vi "harmony_final.vi"() -> ()   [LabVIEW 2017]
uses:
  <vilib>/measure/maspectr.llb/FFT Spectrum (Mag-Phase) for 1 Chan.vi
  <vilib>/Instr/_visa.llb/VISA Configure Serial Port (Instr).vi
  <vilib>/measure/NI_MAPro.lvlib
panel:
  out "Si":bool
  out "Lá":bool
  out "Sol":bool
  out "Fá":bool
  out "Mi":bool
  out "Ré":bool
  out "Dó":bool
  out "Frequências":cluster{"f0":dbl, "df":dbl, "magnitude":dbl[]}(graph)
  out "Frequência":i32
  out "Waveform Chart":waveform(dbl)(graph)
  in  "Reset":bool
  in  "Porta Serial":refnum<visa-resource-name>
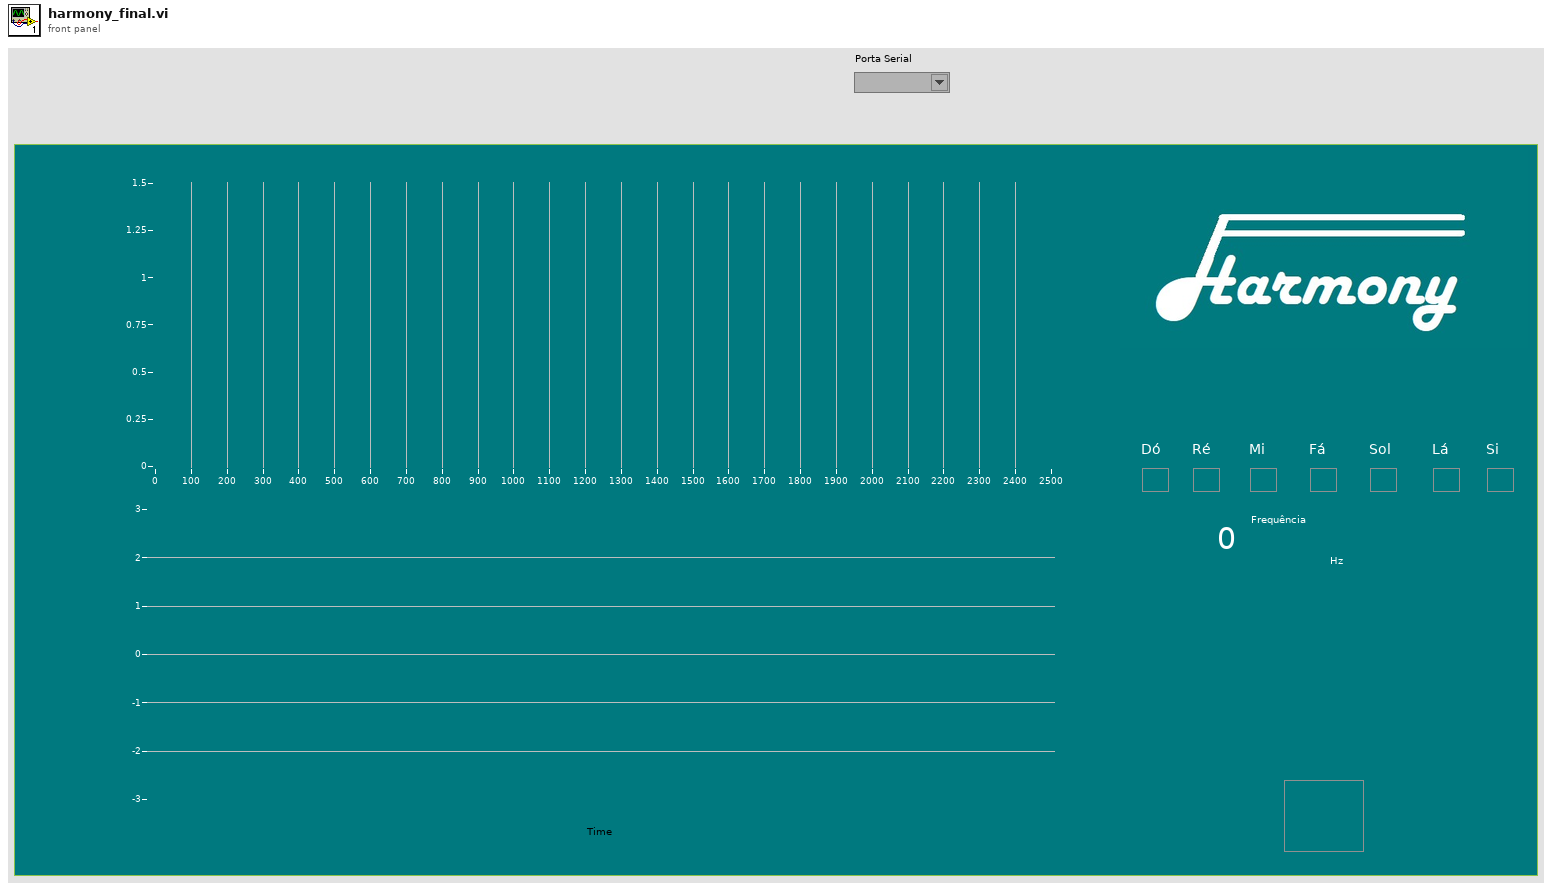
[diagram p1: front panel]
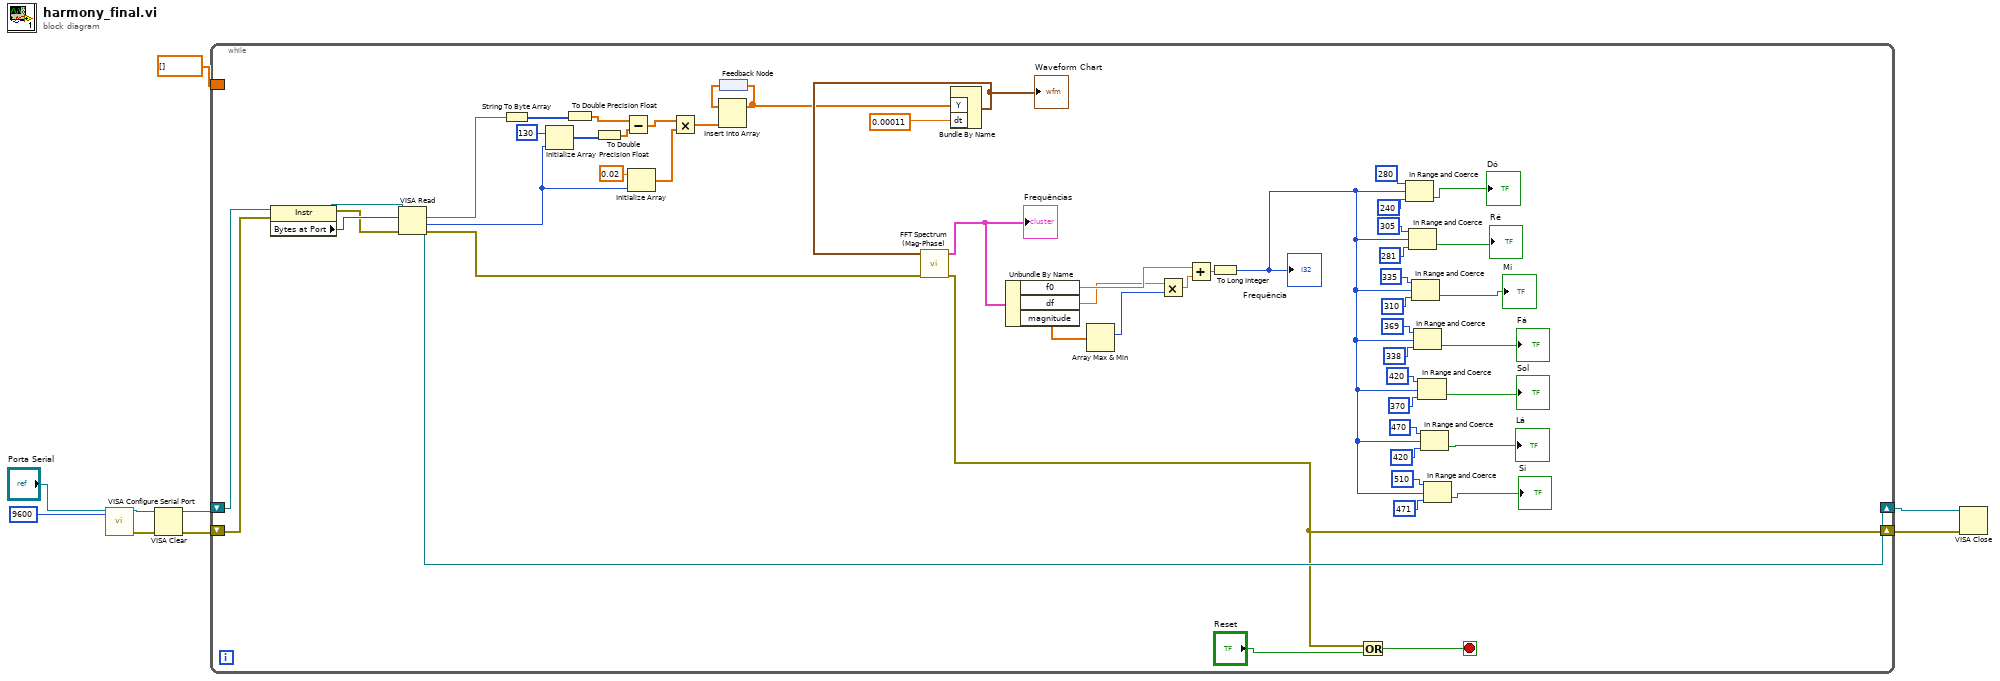
[diagram p0: block diagram]
diagram:
  n1 = call-poly "VISA Configure Serial Port"("VISA resource name"="Porta Serial", "baud rate (9600)"=u32 9600) -> ("VISA resource name out"=w7:refnum<visa-resource-name>, "error out"=w6:errorcluster)  [unwired: 12 in]
  n2 = VISA Clear(VISA resource name=w7, error in (no error)=w6) -> (VISA resource name out=w5:refnum<visa-resource-name>, error out=w4:errorcluster)
  n3 = while {
    shift-right: [w58] -> w3
    shift-left: w5 -> [w63]
    shift-right: [w34] -> w2
    shift-left: w4 -> [w62]
    border: dbl[] [] -> [_]
    stop <- w54 stop-if-true
    n4 = property class="Instr"(reference=w63, error in=w62) -> (reference out=w60:refnum<visa-resource-name>, error out=w59:errorcluster, "Bytes at Port"=w61:u32)
    n5 = VISA Read(VISA resource name=w60, byte count=w61, error in (no error)=w59) -> (VISA resource name out=w58:refnum<visa-resource-name>, read buffer=w56:string, return count=w44:u32, error out=w37:errorcluster)
    n6 = String To Byte Array(string=w56) -> (unsigned byte array=w51:u8[])
    n7 = Initialize Array(130, w44) -> (w46:i32[])
    n8 = To Double Precision Float(number=w51) -> (double precision float=w50:dbl[])
    n9 = To Double Precision Float(number=w46) -> (double precision float=w45:dbl[])
    n10 = Subtract(x=w50, y=w45) -> (x-y=w49:dbl[])
    n11 = Initialize Array(0.02, w44) -> (w42:dbl[])
    n12 = Multiply(x=w49, y=w42) -> (x*y=w48:dbl[])
    n13 = feedback #1() -> (w57:dbl[])
    n14 = Insert Into Array(array=w57, new element=w48) -> (w10:dbl[])  [unwired: 1 in]
    n15 = feedback-in #1(w10) -> ()
    n16 = Bundle By Name("Y"=w10, "dt"=0.00011) -> (w53:waveform(dbl))  [unwired: 1 in]
    "Waveform Chart" <- w53
    n17 = call-poly <vilib>:"FFT Spectrum (Mag-Phase).vi"("error in (no error)"=w37, "time signal"=w53) -> ("error out"=w34:errorcluster, "magnitude"=w52:cluster{"f0":dbl, "df":dbl, "magnitude":dbl[]})  [unwired: 5 in, 3 out]
    "Frequências" <- w52
    n18 = Unbundle By Name(w52) -> ("f0"=w39:dbl, "df"=w38:dbl, "magnitude"=w36:dbl[])
    n19 = Array Max & Min(array=w36) -> (max index (indices)=w35:i32)  [unwired: 3 out]
    n20 = Multiply(x=w38, y=w35) -> (x*y=w40:dbl)
    n21 = Add(x=w39, y=w40) -> (x+y=w41:dbl)
    n22 = To Long Integer(number=w41) -> (32bit integer=w18:i32)
    "Frequência" <- w18
    n23 = Or(x=w34, y="Reset") -> (x .or. y?=w54:bool)
    n24 = In Range and Coerce(upper limit=280, x=w18, lower limit=240) -> (In Range?=→"Dó":bool)  [unwired: 1 out]
    n25 = In Range and Coerce(upper limit=305, x=w18, lower limit=281) -> (In Range?=→"Ré":bool)  [unwired: 1 out]
    n26 = In Range and Coerce(upper limit=335, x=w18, lower limit=310) -> (In Range?=→"Mi":bool)  [unwired: 1 out]
    n27 = In Range and Coerce(upper limit=369, x=w18, lower limit=338) -> (In Range?=→"Fá":bool)  [unwired: 1 out]
    n28 = In Range and Coerce(upper limit=420, x=w18, lower limit=370) -> (In Range?=→"Sol":bool)  [unwired: 1 out]
    n29 = In Range and Coerce(upper limit=470, x=w18, lower limit=420) -> (In Range?=→"Lá":bool)  [unwired: 1 out]
    n30 = In Range and Coerce(upper limit=510, x=w18, lower limit=471) -> (In Range?=→"Si":bool)  [unwired: 1 out]
  }
  n31 = VISA Close(VISA resource name=w3, error in (no error)=w2) -> ()  [unwired: 1 out]
